vi "VCI_OpenDevice.vi"() -> (2 "DevIndex":u32, 3 "DevType":u32, 5 "VCI_OpenDevice":u32)   [LabVIEW 2014]
uses:
  ControlCAN.dll
panel:
  out "Reserved":u32
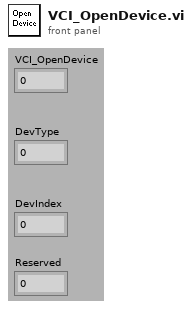
[diagram p1: front panel]
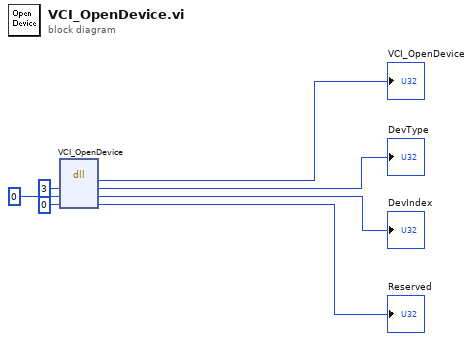
[diagram p0: block diagram]
diagram:
  n1 = dll-call lib="PTH22abs D\tDocuments\tCan总线canControlCAN.dll" fn="VCI_OpenDevice"("DevType"=u32 3, "DevIndex"=u32 0, "Reserved"=u32 0) -> ("VCI_OpenDevice"=→"VCI_OpenDevice":u32, "DevType"=→"DevType":u32, "DevIndex"=→"DevIndex":u32, "Reserved"=→"Reserved":u32)  [unwired: 3 in, 2 out]
